vi "Read.vi"(8 "error in (no error)":errorcluster, 9 "Text to prepend to sentence":string="\n", 10 "Minimum Number of Messages (1)":i32=1, 11 "VISA resource name":refnum<visa-resource-name>) -> (0 "error out":errorcluster, 1 "Remaining Sentence":string, 2 "Ocean Server Sentences":string[](array[string]), 3 "VISA resource name out":refnum<visa-resource-name>)   [LabVIEW 2011, in "Ocean Server OS4000.lvlib"]
doc: "Reads the input buffer and creates a single message received. The common sequence of VIs for obtaining data from the instrument is as follows:\n\n<b>1. Fetch Data\n2. Get Sentence Type\n3. Parse Sentence</b>"
uses:
  Ocean Server OS4000.lvlib
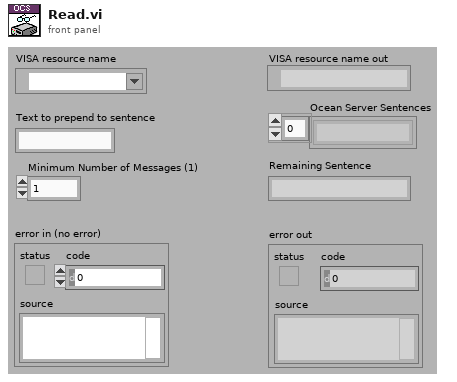
[diagram p1: front panel]
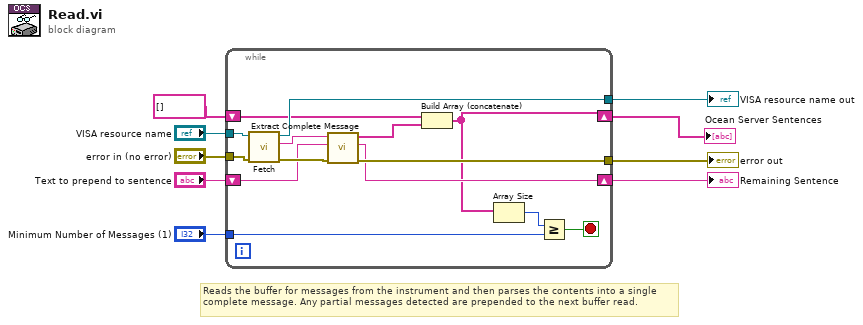
[diagram p0: block diagram]
diagram:
  # "Reads the buffer for messages from the instrument and then parses the contents into a single complete message. Any partial messages detected are prepended to the next buffer read."
  n1 = while {
    tunnel: "VISA resource name" -> [w23]
    tunnel: "error in (no error)" -> [w22]
    tunnel: [w20] -> w7
    tunnel: [w18] -> w5
    shift-right: [w16] -> w6
    shift-left: "Text to prepend to sentence" -> [w17]
    tunnel: "Minimum Number of Messages (1)" -> [w14]
    shift-right: [w12] -> w2
    shift-left: string[] [] ("array") -> [w10]
    stop <- w11 stop-if-true
    n2 = call "Fetch.vi"("error in (no error)"=w22, "VISA resource name"=w23) -> ("error out"=w21:errorcluster, "Read Buffer"=w19:string, "VISA resource name out"=w18:refnum<visa-resource-name>)  [unwired: 5 in]
    n3 = call "Extract Complete Message.vi"("Error in (no error)"=w21, "Text to prepend to messages"=w17, "String of Instrument Messages"=w19) -> ("Error out"=w20:errorcluster, "Remaining String"=w16:string, "Ocean Server Sentences"=w13:string[])  [unwired: 6 in]
    n4 = Build Array (concatenate)(w10, w13) -> (w12:string[])
    n5 = Array Size(array=w12) -> (size(s)=w15:i32)
    n6 = Greater Or Equal?(x=w15, y=w14) -> (x >= y?=w11:bool)
  }
  "Remaining Sentence" <- w6
  "error out" <- w7
  "VISA resource name out" <- w5
  "Ocean Server Sentences" <- w2
